vi "Test Get In Public Documents.vi"() -> ()   [LabVIEW 2021, in "Path Utilities.lvlib"]
doc: "Unit Test for \"Get In Public Documents.vi\"."
uses:
  Path Utilities.lvlib
panel:
  out "error out":errorcluster
  out "Pass - System Path with Base":bool
  out "Result - System Path with Base":path
  out "Expected - System Path with Base":path
  out "Pass - System Path Only":bool
  out "Result - System Path Only":path
  out "Expected - System Path Only":path
  in  "Base Path":path=path "Company/Application"
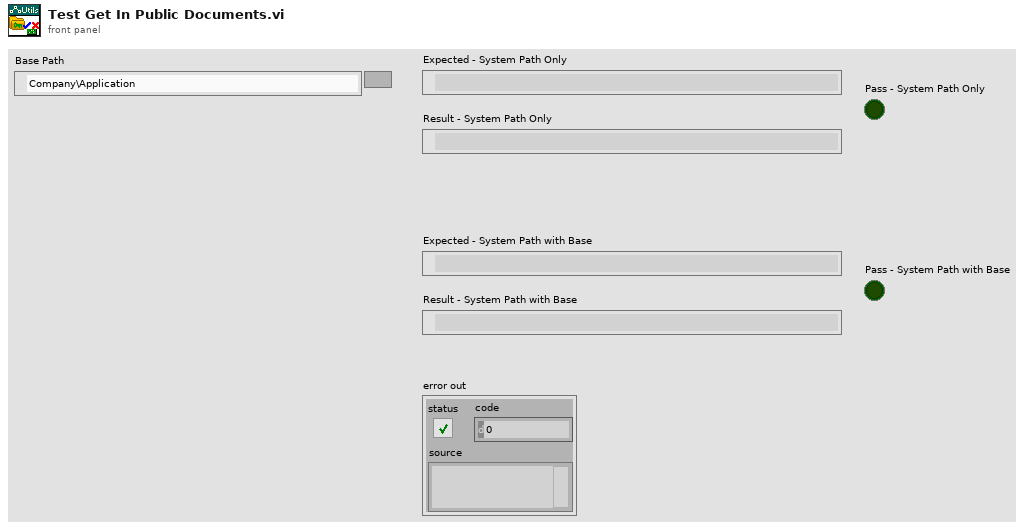
[diagram p1: front panel]
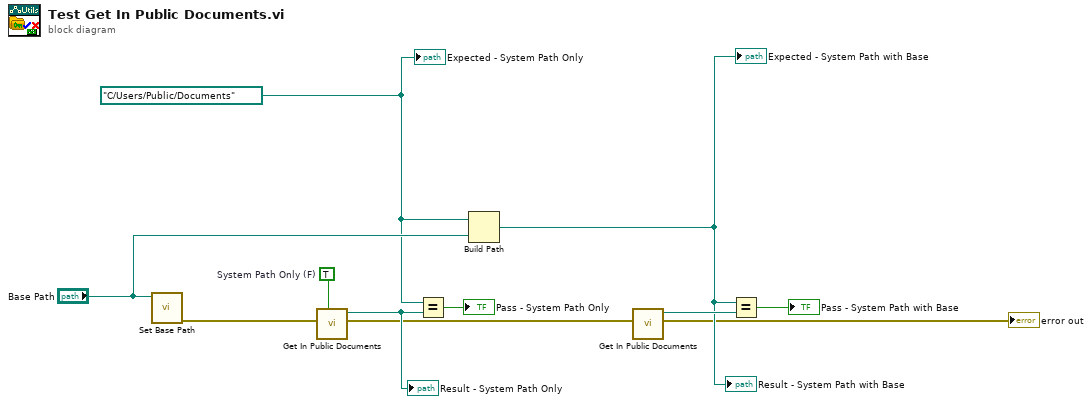
[diagram p0: block diagram]
diagram:
  w1 = path "C:/Users/Public/Documents" ("base path")
  w10 = TRUE  # System Path Only (F)
  n1 = call "Set Base Path.vi"("Base Path"="Base Path") -> ("error out"=w11:errorcluster)  [unwired: 10 in]
  n2 = call "Get In Public Documents.vi"("System Path Only (F)"=w10, "error in (no error)"=w11) -> ("error out"=w7:errorcluster, "Path"=w8:path)  [unwired: 8 in]
  "Result - System Path Only" <- w8
  n3 = Equal?(x=w1, y=w8) -> (x = y?=→"Pass - System Path Only":bool)
  n4 = Build Path(base path=w1, name or relative path="Base Path") -> (appended path=w3:path)
  "Expected - System Path with Base" <- w3
  "Result - System Path with Base" <- w3
  n5 = call "Get In Public Documents.vi"("error in (no error)"=w7) -> ("error out"=→"error out":errorcluster, "Path"=w5:path)  [unwired: 9 in]
  n6 = Equal?(x=w3, y=w5) -> (x = y?=→"Pass - System Path with Base":bool)
  "Expected - System Path Only" <- w1
